vi "GOOP_ProviderClasses_SortingDialog.vi"(8 "error in (no error)":errorcluster) -> (0 "error out":errorcluster, 2 "Cancelled":bool, 3 "FirstProvider":string)   [LabVIEW 2020]
panel:
  in  "Cancel":bool
  in  "Save":bool
  in  "Down":bool
  in  "Up":bool
  in  "ClassProviders":i32(listbox) caption="Class Providers Order"
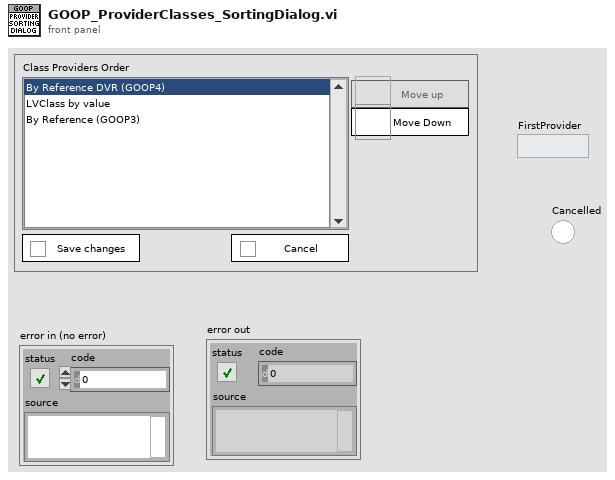
[diagram p1: front panel]
types:
  T1 = cluster{"Providers":cluster{"Provider":string, "Active":bool, "TranslatedName":string}[], "Provider":string}
  T2 = cluster{"Provider":string, "Active":bool, "TranslatedName":string}
  T3 = enum8{"Enabled", "Disabled", "Disabled and Grayed Out"}
  T4 = cluster{"Provider":string, "Active":bool, "TranslatedName":string}[]
  T5 = typedef "LVPoint32TypeDef.ctl" = cluster{"Horizontal":i32, "Vertical":i32}
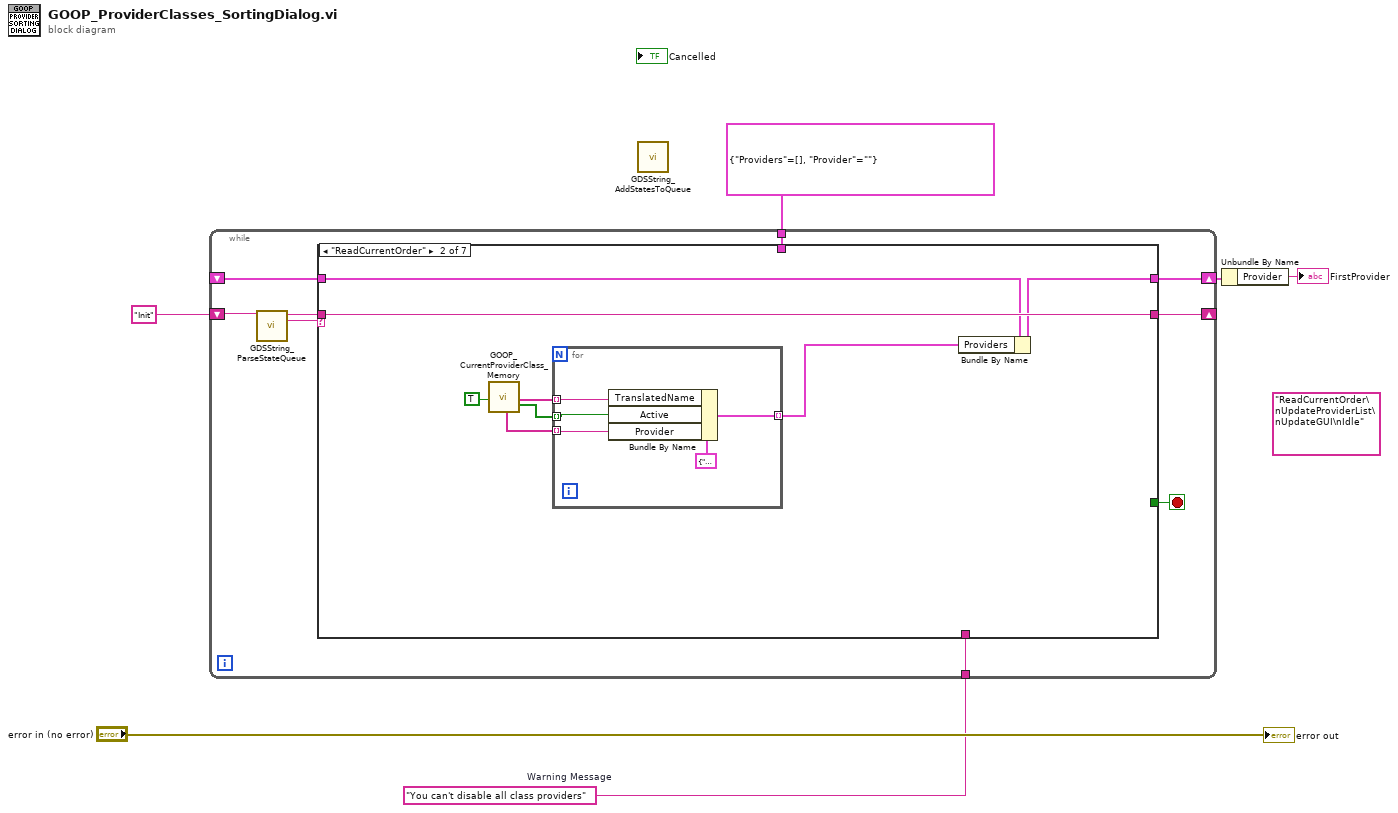
[diagram p0: block diagram]
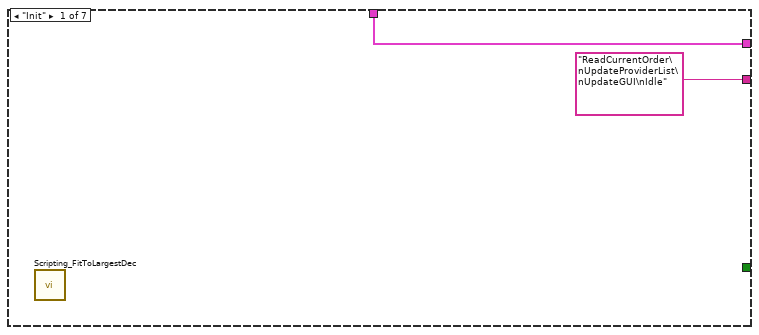
[diagram p2: hidden frame]
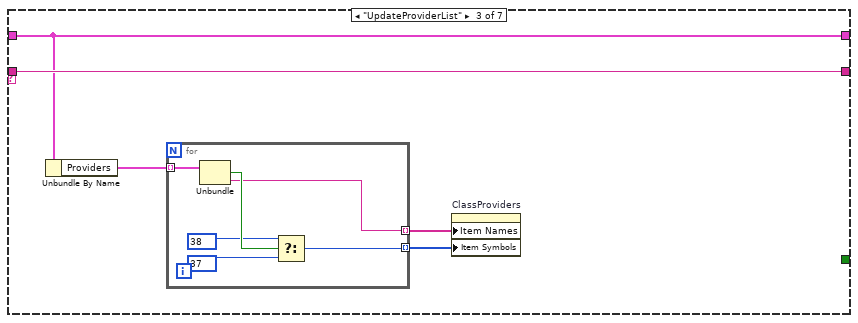
[diagram p3: hidden frame]
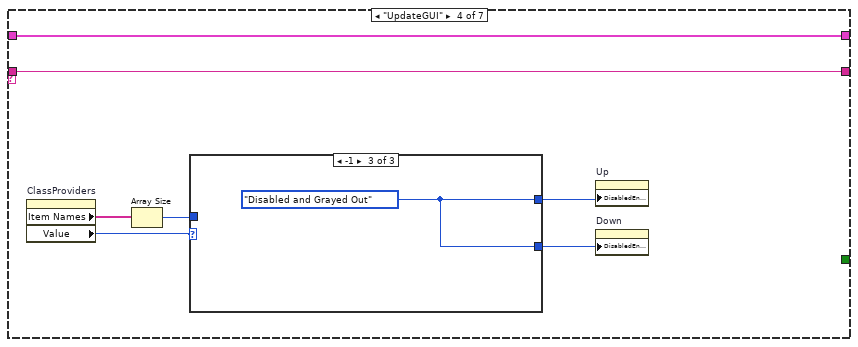
[diagram p4: hidden frame]
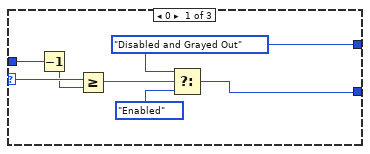
[diagram p5: hidden frame]
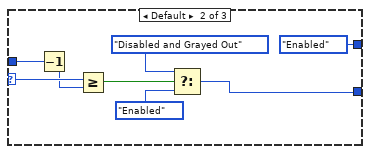
[diagram p6: hidden frame]
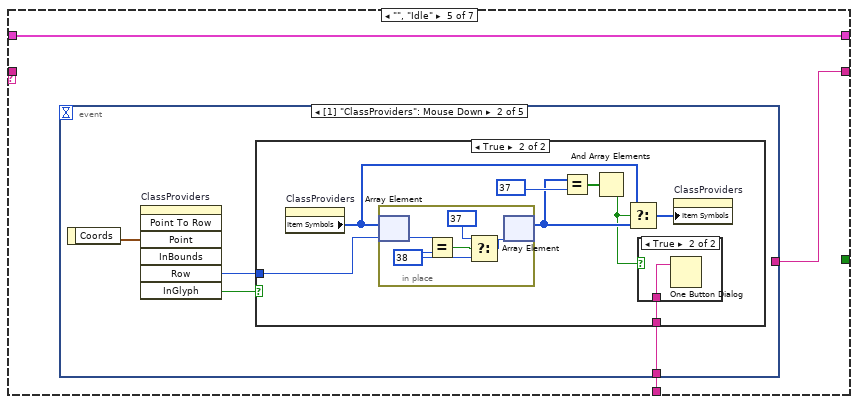
[diagram p7: hidden frame]
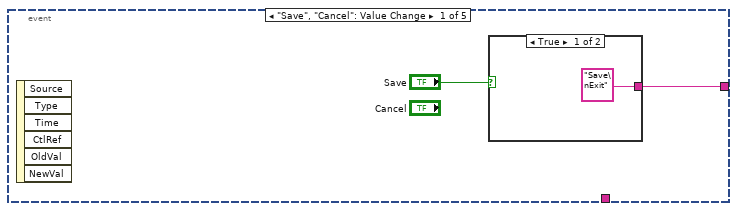
[diagram p8: hidden frame]
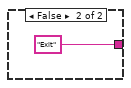
[diagram p9: hidden frame]
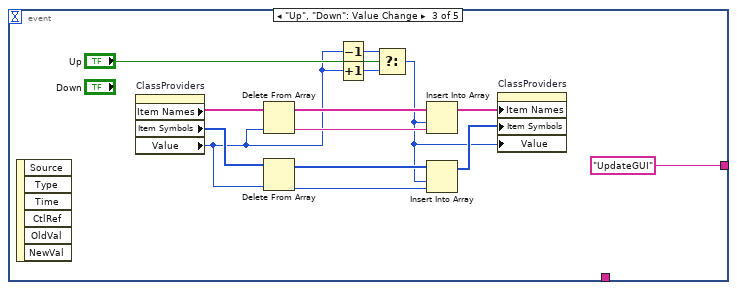
[diagram p12: hidden frame]
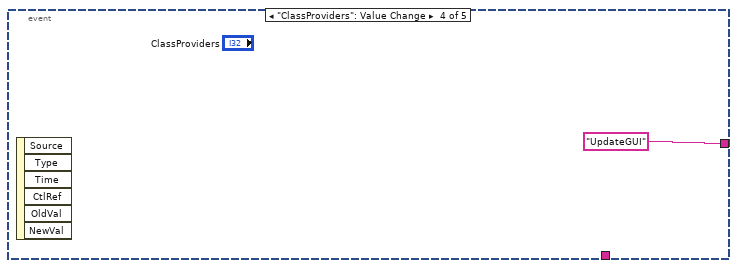
[diagram p13: hidden frame]
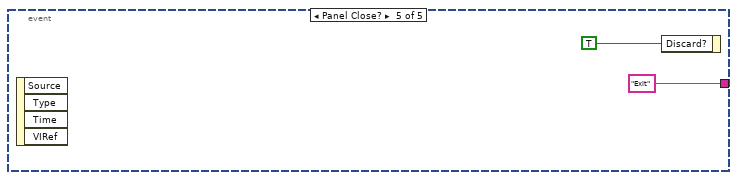
[diagram p14: hidden frame]
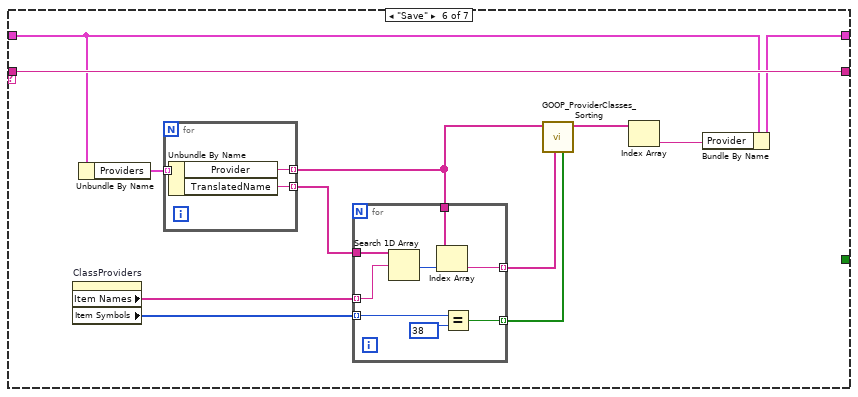
[diagram p15: hidden frame]
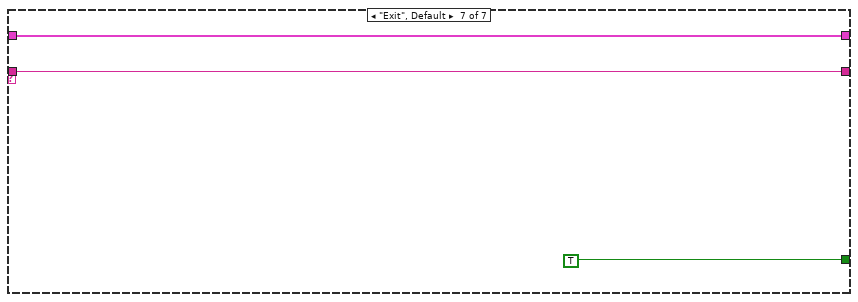
[diagram p16: hidden frame]
diagram:
  (unwired) "ReadCurrentOrder\nUpdateProviderList\nUpdateGUI\nIdle" ("Remaining States")
  w3 = "You can't disable all class providers"  # Warning Message
  n1 = while {
    shift-right: [w13] -> _
    shift-left: "Init" -> [w14]
    tunnel: T1 {"Providers"=[], "Provider"=""} -> [w10]
    shift-right: [w9] -> w2
    shift-left: _ -> [w8]
    tunnel: w3 -> [w7]
    stop <- w15 stop-if-true
    n2 = call <resource>:"GDSString_ParseStateQueue.vi"("State Queue"=w14) -> ("Remaining States"=w11:string, "Current State"=w12:string)  [unwired: 10 in, 3 out]
    n3 = case shown="\"ReadCurrentOrder\"" w12 {
      tunnel: [_ _ _ _ _ _ TRUE] -> w15
      tunnel: ["ReadCurrentOrder\nUpdateProviderList\nUpdateGUI\nIdle" ("Remaining States") w25 w35 w48 w67 w118 w131] -> w13
      tunnel: w11 -> [_ w25 w35 w48 _ w118 w131]
      tunnel: [w17 w23 w34 w47 w66 w109 w130] -> w9
      tunnel: w10 -> [w17 _ _ _ _ _ _]
      tunnel: w8 -> [_ w24 w34 w47 w66 w117 w130]
      tunnel: w7 -> [_ _ _ _ w65 _ _]
      frame "Init" {
        n4 = call <resource>:"Scripting_FitToLargestDec.vi"() -> ()  [unwired: 6 in, 2 out]
      }
      frame "ReadCurrentOrder" {
        n5 = call <resource>:"GOOP_CurrentProviderClass_Memory.vi"("IgnoreFilter(False)"=TRUE) -> ("AllClassProviders(OriginalNames)"=w21:string[], "AllClassProviders(TranslatedNames)"=w20:string[], "AllClassProvidersFilterSettings"=w19:bool[])  [unwired: 12 in, 4 out]
        n6 = for {
          tunnel: w21 -> [w27] mode=indexing
          tunnel: w20 -> [w29] mode=indexing
          tunnel: w19 -> [w28] mode=indexing
          tunnel: [w26] -> w18 mode=indexing
          n7 = Bundle By Name(cluster=T2 {"Provider"="", "Active"=FALSE, "TranslatedName"=""} ("Cluster"), "TranslatedName"=w29, "Active"=w28, "Provider"=w27) -> (w26:T2)
        }
        n8 = Bundle By Name(cluster=w24, "Providers"=w18) -> (w23:T1)
      }
      frame "UpdateProviderList" {
        n9 = Unbundle By Name(w34) -> ("Providers"=w33:T4)
        n10 = for {
          tunnel: w33 -> [w41] mode=indexing
          tunnel: [w37] -> w31 mode=indexing
          tunnel: [w36] -> w32 mode=indexing
          n11 = Unbundle(w41) -> ("Active"=w40:bool, "TranslatedName"=w36:string)  [unwired: 1 out]
          n12 = Select(t=38, s=w40, f=37) -> (s? t:f=w37:i32)
        }
        n13 = property on="ClassProviders" class="LstBox (strict)"("Item Names"=w32, "Item Symbols"=w31) -> ()  [unwired: 2 in, 2 out]
      }
      frame "UpdateGUI" {
        n14 = property on="ClassProviders" class="LstBox (strict)"() -> ("Item Names"=w43:string[], "Value"=w46:i32)  [unwired: 2 in, 2 out]
        n15 = Array Size(array=w43) -> (size(s)=w42:i32)
        n16 = case shown="-1" w46 {
          selector: w46 -> [w55 w63 _]
          tunnel: [w50 T3."Enabled" ("Disabled") w64] -> w45
          tunnel: [w51 w59 w64] -> w44
          tunnel: w42 -> [w54 w62 _]
          frame 0 {
            w50 = T3."Disabled and Grayed Out" ("Disabled")
            n17 = Decrement(x=w54) -> (x-1=w53:i32)
            n18 = Greater Or Equal?(x=w55, y=w53) -> (x >= y?=w52:bool)
            n19 = Select(t=w50, s=w52, f=T3."Enabled" ("Disabled")) -> (s? t:f=w51:T3)
          }
          frame Default {
            n20 = Decrement(x=w62) -> (x-1=w61:i32)
            n21 = Greater Or Equal?(x=w63, y=w61) -> (x >= y?=w60:bool)
            n22 = Select(t=T3."Disabled and Grayed Out" ("Disabled"), s=w60, f=T3."Enabled" ("Disabled")) -> (s? t:f=w59:T3)
          }
          frame -1 {
            w64 = T3."Disabled and Grayed Out" ("Disabled")
          }
        }
        n23 = property on="Up" class="Bool"("DisabledEnum"=w45) -> ()  [unwired: 2 in, 2 out]
        n24 = property on="Down" class="Bool"("DisabledEnum"=w44) -> ()  [unwired: 2 in, 2 out]
      }
      frame "", "Idle" {
        n25 = event shown="[1] \"ClassProviders\": Mouse Down" {
          selector: _ -> [_ _ _ _ _]
          dyn-events: _ -> [_ _ _ _ _]
          timeout: _ -> [_ _ _ _ _]
          tunnel: [w69 _ "UpdateGUI" "UpdateGUI" "Exit"] -> w67
          tunnel: w65 -> [_ w72 _ _ _]
          event "Save", "Cancel": Value Change {
            n26 = event-data() -> ()  [unwired: 1 in, 6 out]
            n27 = case shown="True" "Save" {
              tunnel: ["Save\nExit" "Exit"] -> w69
              frame True {
              }
              frame False {
              }
            }
          }
          event "ClassProviders": Mouse Down {
            n28 = event-data() -> ("Coords"=w75:T5)  [unwired: 1 in]
            n29 = invoke on="ClassProviders" class="LstBox (strict)" method="Point To Row"("Point"=w75) -> ("Row"=w73:i32, "InGlyph"=w74:bool)  [unwired: 6 in, 5 out]
            n30 = case shown="True" w74 {
              tunnel: w73 -> [_ w83]
              tunnel: w72 -> [_ w76]
              frame False {
              }
              frame True {
                n31 = property on="ClassProviders" class="LstBox (strict)"() -> ("Item Symbols"=w79:i32[])  [unwired: 2 in, 2 out]
                n32 = in-place {
                  w87 = 38
                  n33 = in-place-array #1(w79, w83) -> (w89:i32)
                  n34 = Equal?(x=w89, y=w87) -> (x = y?=w88:bool)
                  n35 = Select(t=37, s=w88, f=w87) -> (s? t:f=w85:i32)
                  n36 = in-place-array #1(w85) -> (w80:i32[])  [unwired: 1 out]
                }
                n37 = Equal?(x=w80, y=37) -> (x = y?=w81:bool[])
                n38 = And Array Elements(Boolean array=w81) -> (logical AND=w77:bool)
                n39 = Select(t=w79, s=w77, f=w80) -> (s? t:f=w78:i32[])
                n40 = case shown="True" w77 {
                  tunnel: w76 -> [_ w84]
                  frame False {
                  }
                  frame True {
                    n41 = One Button Dialog(message=w84) -> ()  [unwired: 1 in, 1 out]
                  }
                }
                n42 = property on="ClassProviders" class="LstBox (strict)"("Item Symbols"=w78) -> ()  [unwired: 2 in, 2 out]
              }
            }
          }
          event "Up", "Down": Value Change {
            n43 = event-data() -> ()  [unwired: 1 in, 6 out]
            n44 = property on="ClassProviders" class="LstBox (strict)"() -> ("Item Names"=w102:string[], "Item Symbols"=w101:i32[], "Value"=w92:i32)  [unwired: 2 in, 2 out]
            n45 = Delete From Array(array=w102, index=w92) -> (deleted portion=w98:string, array with subset deleted=w100:string[])  [unwired: 1 in]
            n46 = Delete From Array(array=w101, index=w92) -> (deleted portion=w97:i32, array with subset deleted=w99:i32[])  [unwired: 1 in]
            n47 = Decrement(x=w92) -> (x-1=w91:i32)
            n48 = Increment(x=w92) -> (x+1=w90:i32)
            n49 = Select(t=w91, s="Up", f=w90) -> (s? t:f=w93:i32)
            n50 = Insert Into Array(array=w100, index=w93, new element=w98) -> (w95:string[])
            n51 = Insert Into Array(array=w99, index=w93, new element=w97) -> (w94:i32[])
            n52 = property on="ClassProviders" class="LstBox (strict)"("Item Names"=w95, "Item Symbols"=w94, "Value"=w93) -> ()  [unwired: 2 in, 2 out]
          }
          event "ClassProviders": Value Change {
            n53 = event-data() -> ()  [unwired: 1 in, 6 out]
          }
          event Panel Close? {
            n54 = event-data() -> ()  [unwired: 1 in, 4 out]
            n55 = event-data("Discard?"=TRUE) -> ()  [unwired: 1 in, 1 out]
          }
        }
      }
      frame "Save" {
        n56 = property on="ClassProviders" class="LstBox (strict)"() -> ("Item Names"=w114:string[], "Item Symbols"=w112:i32[])  [unwired: 2 in, 2 out]
        n57 = Unbundle By Name(w117) -> ("Providers"=w116:T4)
        n58 = for {
          tunnel: w116 -> [w129] mode=indexing
          tunnel: [w128] -> w107 mode=indexing
          tunnel: [w127] -> w115 mode=indexing
          n59 = Unbundle By Name(w129) -> ("Provider"=w128:string, "TranslatedName"=w127:string)
        }
        n60 = for {
          tunnel: w115 -> [w126]
          tunnel: w114 -> [w125] mode=indexing
          tunnel: w107 -> [w124]
          tunnel: [w122] -> w113 mode=indexing
          tunnel: w112 -> [w121] mode=indexing
          tunnel: [w119] -> w111 mode=indexing
          n61 = Search 1D Array(1D array=w126, element=w125) -> (index of element=w123:i32)  [unwired: 1 in]
          n62 = Index Array(array=w124, index=w123) -> (element=w122:string)
          n63 = Equal?(x=w121, y=38) -> (x = y?=w119:bool)
        }
        n64 = call <resource>:"GOOP_ProviderClasses_Sorting.vi"("ProvidersClassesActive"=w111, "ProvidersClassesSortOrder"=w113, "AllClassProvidersIn(OriginalNames)"=w107) -> ("AllClassProvidersOut(OriginalNames)"=w110:string[])  [unwired: 6 in, 2 out]
        n65 = Index Array(array=w110) -> (element=w108:string)  [unwired: 1 in]
        n66 = Bundle By Name(cluster=w117, "Provider"=w108) -> (w109:T1)
      }
      frame "Exit", Default {
      }
    }
  }
  n67 = call <resource>:"GDSString_AddStatesToQueue.vi"() -> ()  [unwired: 15 in, 1 out]
  n68 = Unbundle By Name(w2) -> ("Provider"=→"FirstProvider":string)
  "error out" <- "error in (no error)"
